vi "test.vi"() -> ()   [LabVIEW 2016]
uses:
  TCPServer/TCPServer.lvclass
  C:/Users/aanania/Documents/ts_monochromator_windows/ts_labview_tcp/TCPCommunicator/TCPCommunicator.lvclass
  TCPComEvents/TCPComEvents.lvclass/TCPComEvents.ctl
  TCPCommunicator/TCPCommunicator.lvclass/TCPCommunicator.ctl
  TCPCommunicator/TCPCommunicator.lvclass
  TCPComEvents/TCPComEvents.lvclass
panel:
  out "error out":errorcluster
  out "message received":string
  in  "stop":bool
  in  "Send":bool
  in  "Message":string="test"
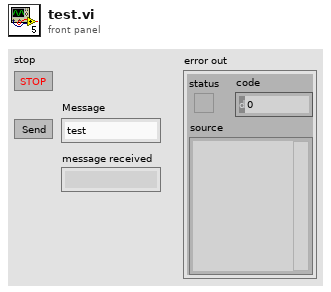
[diagram p1: front panel]
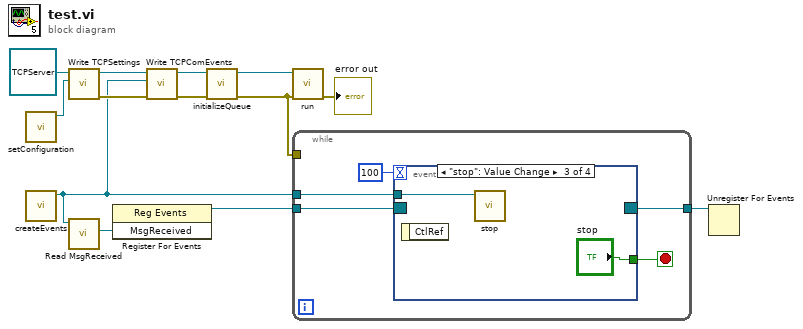
[diagram p0: block diagram]
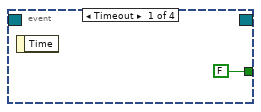
[diagram p2: hidden frame]
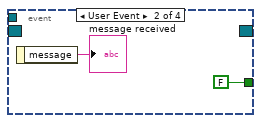
[diagram p3: hidden frame]
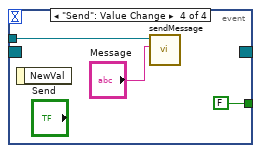
[diagram p4: hidden frame]
diagram:
  n1 = call "setConfiguration.vi"() -> ("TCPSettings out"=w12:refnum<class "TCPSettings.lvclass">)  [unwired: 11 in]
  n2 = call "createEvents.vi"() -> ("TCPComEvents out"=w7:refnum<class "TCPComEvents.lvclass">)  [unwired: 10 in, 1 out]
  n3 = call-dynamic "Write TCPSettings.vi"("TCPSettings.lvclass"=w12, "TCPCommunicator in"=refnum<class "TCPServer.lvclass"> refnum ("TCPServer.lvclass")) -> ("error out"=w10:errorcluster, "TCPCommunicator out"=w11:refnum<class "TCPServer.lvclass">)  [unwired: 8 in]
  n4 = call "Read MsgReceived.vi"("TCPComEvents in"=w7) -> ("MsgReceived"=w8:refnum<user-event>)  [unwired: 8 in, 2 out]
  n5 = register-events(w8) -> (reference out=w9:refnum<event-registration>)  [unwired: 2 in, 1 out]
  n6 = call "Write TCPComEvents.vi"("error in (no error)"=w10, "TCPComEvents.lvclass"=w7, "TCPCommunicator in"=w11) -> ("error out"=w4:errorcluster, "TCPCommunicator out"=w3:refnum<class "TCPServer.lvclass">)  [unwired: 7 in]
  n7 = call-dynamic "initializeQueue.vi"("error in (no error)"=w4, "TCPCommunicator in"=w3) -> ("error out"=w1:errorcluster, "TCPCommunicator out"=w2:refnum<class "TCPServer.lvclass">)  [unwired: 8 in]
  n8 = call "run.vi"("error in (no error)"=w1, "TCPServer in"=w2) -> ("error out"=→"error out":errorcluster)  [unwired: 8 in, 1 out]
  n9 = while {
    tunnel: w9 -> [w18]
    tunnel: w7 -> [w17]
    tunnel: w1 -> [_]
    tunnel: [w14] -> w6
    stop <- w16 stop-if-true
    n10 = event shown="[2] \"stop\": Value Change" {
      selector: w18 -> [_ _ _ _]
      dyn-events: [_ _ _ _] -> w14
      timeout: 100 -> [_ _ _ _]
      tunnel: w17 -> [_ _ w23 w24]
      tunnel: [FALSE ("stop") FALSE ("stop") "stop" FALSE ("stop")] -> w16
      event Timeout {
        n11 = event-data() -> ()  [unwired: 1 in, 1 out]
      }
      event User Event {
        n12 = event-data() -> ("message"=→"message received":string)  [unwired: 1 in]
      }
      event "stop": Value Change {
        n13 = event-data() -> ()  [unwired: 1 in, 1 out]
        n14 = call "stop.vi"("TCPComEvents in"=w23) -> ()  [unwired: 9 in, 2 out]
      }
      event "Send": Value Change {
        n15 = event-data() -> ()  [unwired: 1 in, 1 out]
        n16 = call "sendMessage.vi"("message"="Message", "TCPComEvents in"=w24) -> ()  [unwired: 8 in, 2 out]
      }
    }
  }
  n17 = Unregister For Events(event registration refnum=w6) -> ()  [unwired: 1 in, 1 out]
